vi "InsertBusNumber.vi"(8 "ErrorArray In":errorcluster[](array[cluster]), 10 "BusNumber":i32) -> (0 "ErrorArray Out":errorcluster[](array[cluster]))   [LabVIEW 2014, in "Framework.lvlib"]
uses:
  Framework.lvlib
  <vilib>/Utility/error.llb/Error Cluster From Error Code.vi
  <vilib>/ErrorRing/Error Ring.xnode
  <userlib>/NIST/NISTErrorLib/NISTErrorLib.lvlib
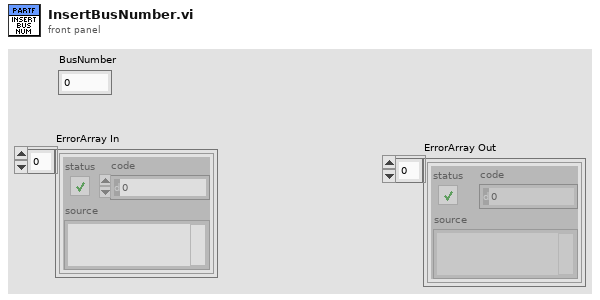
[diagram p1: front panel]
types:
  T1 = typedef "Framework.lvlib/clFrontPanelControlRefs.ctl" = cluster{"TestFilePathRef":refnum<vi>, "BusNumberRef":refnum<vi>, "NumberOfBusesRef":refnum<vi>, "EvtTypeRef":refnum<vi>, "EvtParamsRef":refnum<vi>, "EvtConfigRef":refnum<vi>, "StartTimeRef":refnum<vi>, "EndTimeRef":refnum<vi>, "PmuImpairTypeRef":refnum<vi>, "PmuImpairParamsRef":refnum<vi>, "NetImpairParamsRef":refnum<vi>, "FlagImpairTypeRef":refnum<vi>, "FlagImpairParamsRef":refnum<vi>, "NetImpairTypeRef":refnum<vi>, "OutputFileType":refnum<vi>, "PmuImpairConfigRef":refnum<vi>, "AppTypeRef":refnum<vi>, "ScriptPathRef":refnum<vi>, "ShowPanels?":refnum<vi>}
  T2 = typedef "LVStringsAndValuesArrayTypeDef_U8.ctl" = cluster{"String":string, "Value":u8}[]
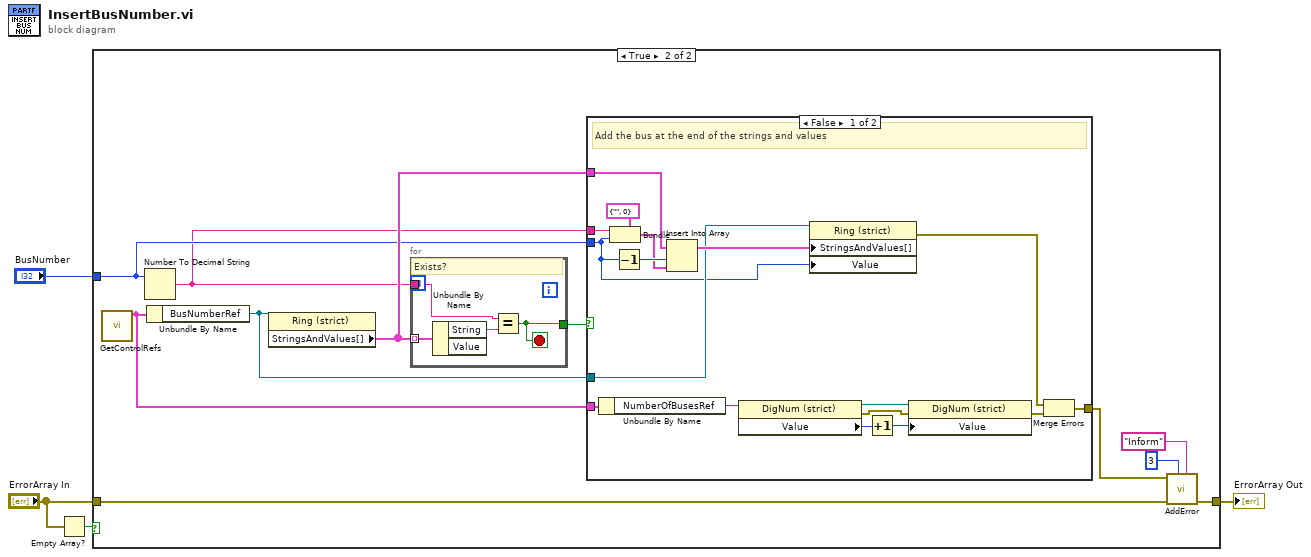
[diagram p0: block diagram]
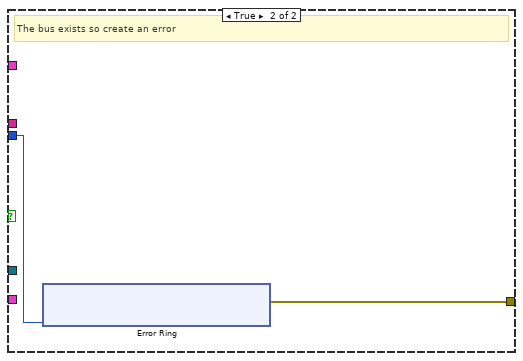
[diagram p3: hidden frame]
diagram:
  n1 = Empty Array?(array="ErrorArray In") -> (empty?=w4:bool)
  n2 = case shown="True" w4 {
    tunnel: "ErrorArray In" -> [w5 w9]
    tunnel: [w5 w8] -> w2
    tunnel: "BusNumber" -> [_ w14]
    frame False {
    }
    frame True {
      n3 = call "GetControlRefs.vi"() -> ("clControlRefs Out"=w12:T1)  [unwired: 11 in]
      n4 = Number To Decimal String(number=w14) -> (decimal integer string=w13:string)  [unwired: 1 in]
      n5 = Unbundle By Name(w12) -> ("BusNumberRef"=w11:refnum<vi>)
      n6 = property class="Ring (strict)"(reference=w11) -> ("StringsAndValues[]"=w15:T2)  [unwired: 1 in, 2 out]
      n7 = for {
        tunnel: w15 -> [w20] mode=indexing
        tunnel: w13 -> [w18]
        tunnel: [w17] -> w16
        stop <- w17 stop-if-true
        # "Exists?"
        n8 = Unbundle By Name(w20) -> ("String"=w19:string)  [unwired: 1 out]
        n9 = Equal?(x=w18, y=w19) -> (x = y?=w17:bool)
      }
      n10 = case shown="False" w16 {
        tunnel: w15 -> [w35 _]
        tunnel: w14 -> [w21 w38]
        tunnel: w13 -> [w36 _]
        tunnel: w12 -> [w32 _]
        tunnel: w11 -> [w26 _]
        tunnel: [w22 w39] -> w10
        frame False {
          # "Add the bus at the end of the strings and values"
          n11 = Unbundle By Name(w32) -> ("NumberOfBusesRef"=w31:refnum<vi>)
          n12 = Bundle(cluster=cluster{"String":string, "Value":u8} {"String"="", "Value"=0} ("element"), "String"=w36, "Value"=w21) -> (w33:cluster{"String":string, "Value":u8})
          n13 = Decrement(x=w21) -> (x-1=w34:i32)
          n14 = Insert Into Array(array=w35, index=w34, new element=w33) -> (w27:T2)
          n15 = property class="DigNum (strict)"(reference=w31) -> (reference out=w29:refnum<vi>, error out=w25:errorcluster, "Value"=w30:u8)  [unwired: 1 in]
          n16 = property class="Ring (strict)"(reference=w26, "StringsAndValues[]"=w27, "Value"=w21) -> (error out=w23:errorcluster)  [unwired: 1 in, 1 out]
          n17 = Increment(x=w30) -> (x+1=w28:u8)
          n18 = property class="DigNum (strict)"(reference=w29, error in=w25, "Value"=w28) -> (error out=w24:errorcluster)  [unwired: 1 out]
          n19 = Merge Errors(w23, w24) -> (w22:errorcluster)
        }
        frame True {
          # "The bus exists so create an error"
          n20 = xnode "Error Ring"("parameter 0"=w38) -> ("error out"=w39:errorcluster)
        }
      }
      n21 = call <userlib>:"AddError.vi"("Severity"="Inform", "Priority"=u8 3, "ErrorArray"=w9, "error in (no error)"=w10) -> ("ErrorArray"=w8:errorcluster[])  [unwired: 6 in, 1 out]
    }
  }
  "ErrorArray Out" <- w2
